vi "RFmxSpecAn Config per Harm & Freq Range (Harms).vi"(0 "SA Handle In":refnum<k21> caption="Instrument Handle In", 1 "# of Harms":u8, 7 "Center Freq (Hz) In":dbl, 11 "error in (no error)":errorcluster, 12 "Read Config File":bool, 13 "Meas Harm #":u8) -> (4 "SA Handle Out":refnum<k21> caption="Instrument Handle Out", 8 "Center Freq (Hz) Out":dbl, 15 "error out":errorcluster)   [LabVIEW 2018]
uses:
  Config Settings.ctl
  <vilib>/Utility/file.llb/Read Delimited Spreadsheet (string).vi
  <resource>/objmgr/RFmxInstr.rc
  <resource>/objmgr/RFmxSpecAn.rc
panel:
  out "Config Settings List":T1[][](array[typedef])
  out "Config Settings":T1
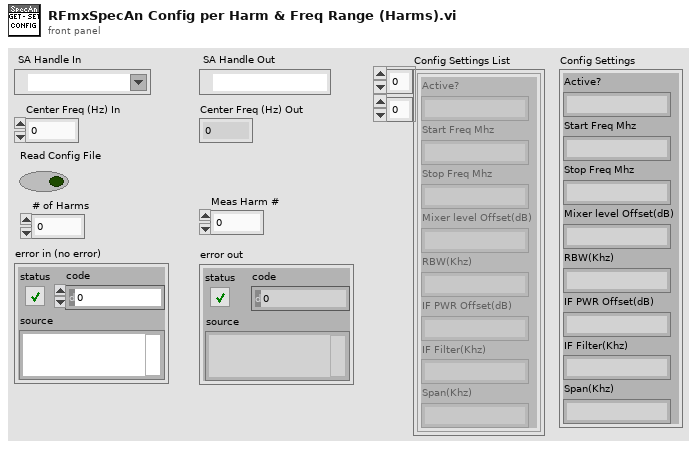
[diagram p1: front panel]
types:
  T1 = typedef "Config Settings.ctl" = cluster{"Active?":string, "Start Freq Mhz":string, "Stop Freq Mhz":string, "Mixer level Offset(dB)":string, "RBW(Khz)":string, "IF PWR Offset(dB)":string, "IF Filter(Khz)":string, "Span(Khz)":string}
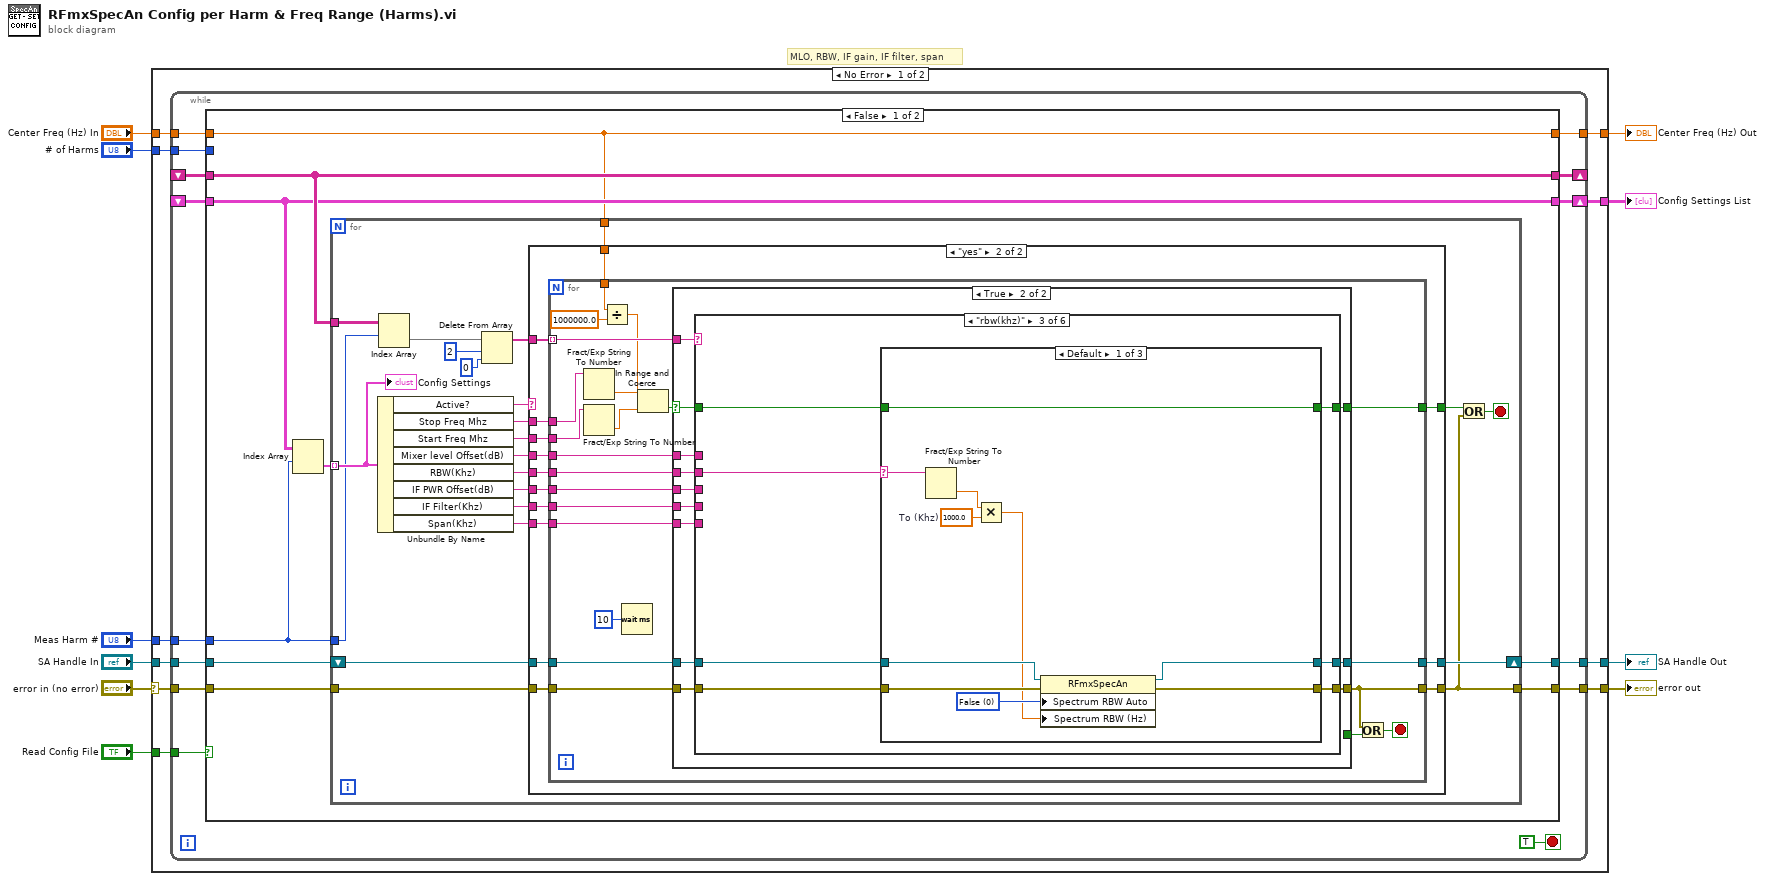
[diagram p0: block diagram]
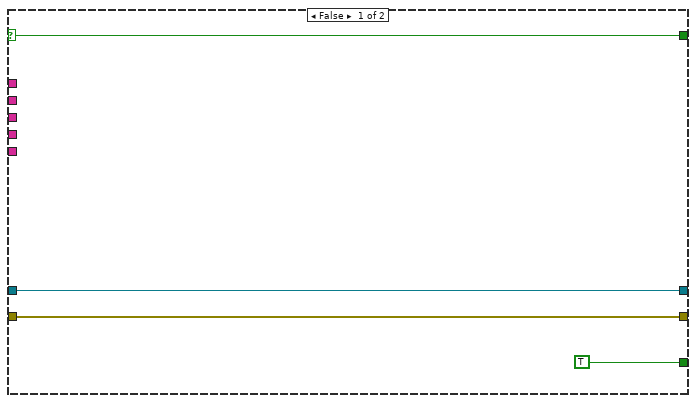
[diagram p3: hidden frame]
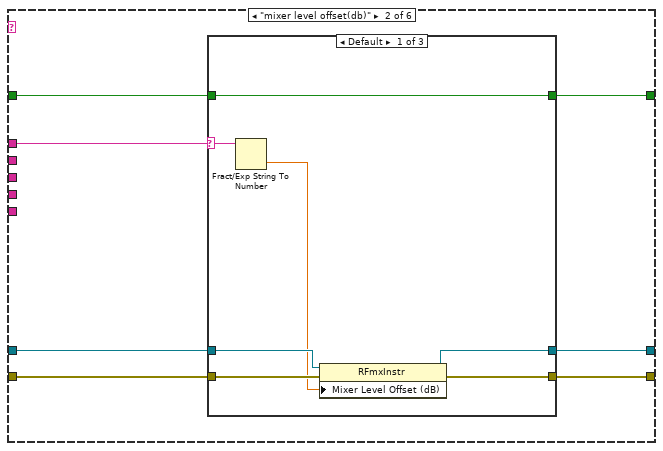
[diagram p5: hidden frame]
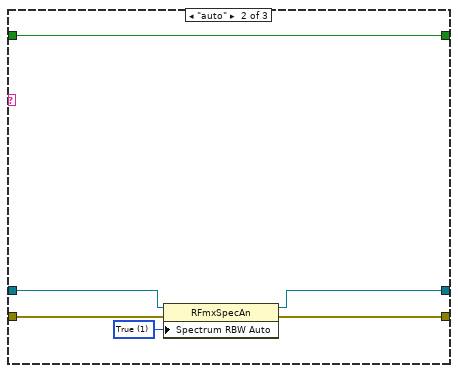
[diagram p8: hidden frame]
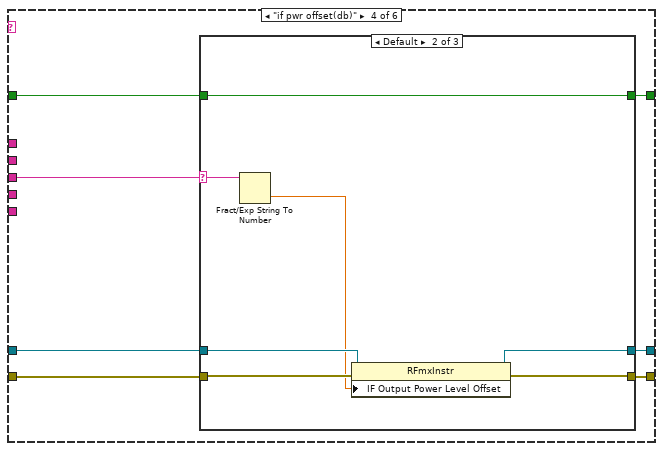
[diagram p10: hidden frame]
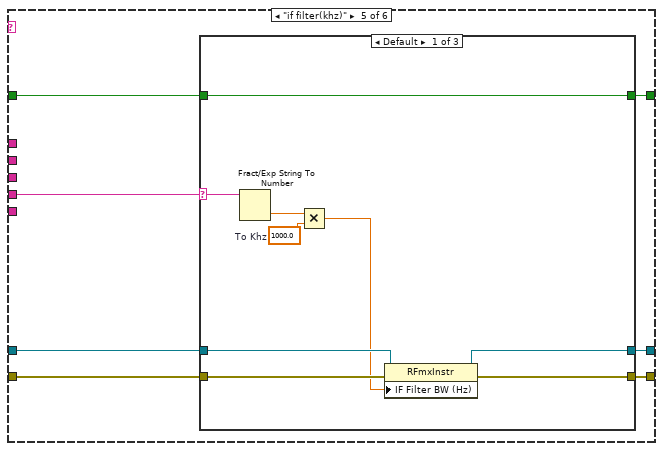
[diagram p13: hidden frame]
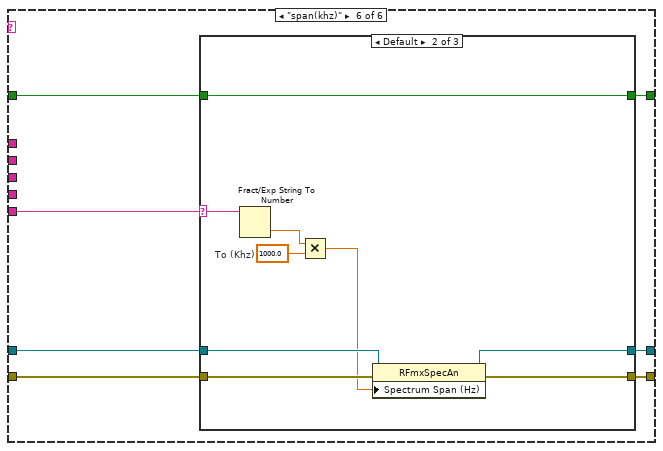
[diagram p16: hidden frame]
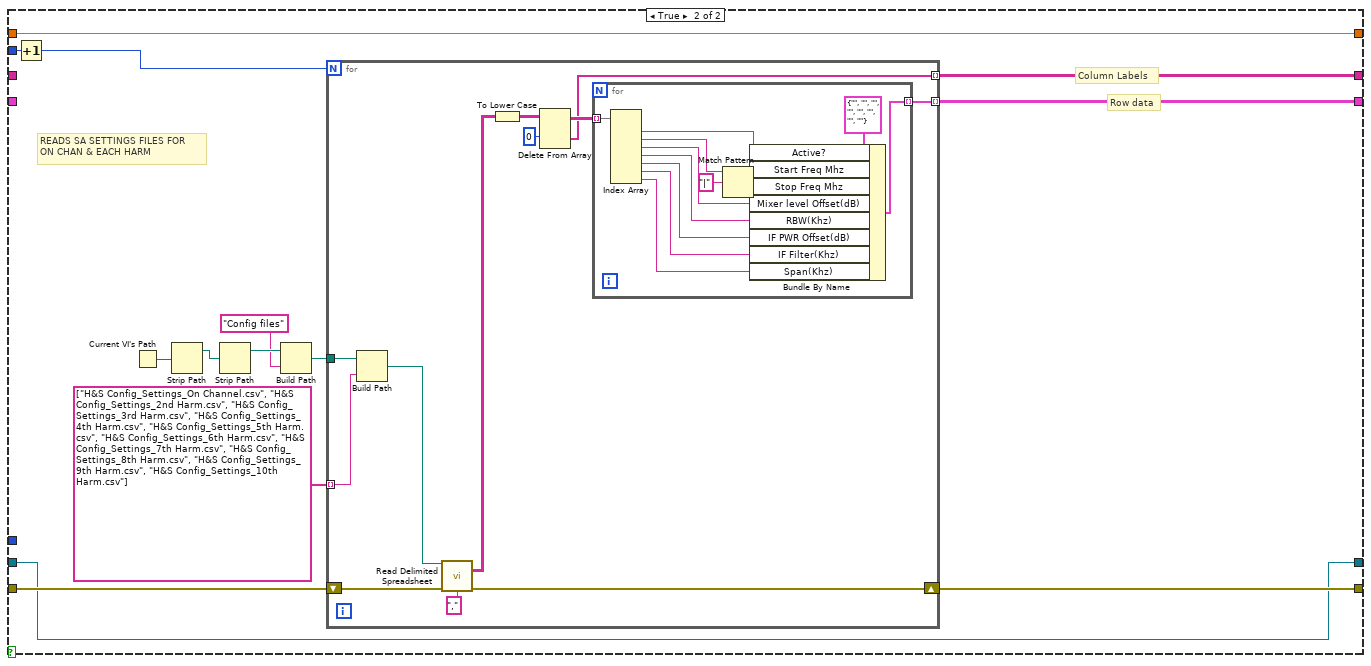
[diagram p19: hidden frame]
diagram:
  # "MLO, RBW, IF gain, IF filter, span"
  n1 = case shown="No Error" "error in (no error)" {
    selector: "error in (no error)" -> [w16 w274]
    tunnel: [w15 w274] -> w2
    tunnel: "SA Handle In" -> [w20 w273]
    tunnel: [w18 w273] -> w1
    tunnel: "Center Freq (Hz) In" -> [w19 w272]
    tunnel: [w17 w272] -> w8
    tunnel: [w14 _] -> w4
    tunnel: "Read Config File" -> [w13 _]
    tunnel: "Meas Harm #" -> [w12 _]
    tunnel: "# of Harms" -> [w11 _]
    frame No Error {
      n2 = while {
        tunnel: w20 -> [w24]
        tunnel: w19 -> [w28]
        tunnel: [w23] -> w18
        tunnel: [w27] -> w17
        tunnel: w16 -> [w33]
        tunnel: [w32] -> w15
        shift-right: [w31] -> w14
        shift-left: _ -> [w29]
        tunnel: w13 -> [w30]
        shift-right: [w26] -> _
        shift-left: _ -> [w25]
        tunnel: w12 -> [w22]
        tunnel: w11 -> [w21]
        stop <- TRUE stop-if-true
        n3 = case shown="False" w30 {
          tunnel: w33 -> [w43 w246]
          tunnel: [w36 w245] -> w32
          tunnel: [w41 w244] -> w31
          tunnel: w29 -> [w41 _]
          tunnel: w28 -> [w40 w243]
          tunnel: [w40 w243] -> w27
          tunnel: [w42 w242] -> w26
          tunnel: w25 -> [w42 _]
          tunnel: w24 -> [w39 w241]
          tunnel: [w35 w241] -> w23
          tunnel: w22 -> [w37 _]
          tunnel: w21 -> [_ w236]
          frame False {
            n4 = Index Array(array=w41, index (row)=w37) -> (element=w38:T1[])  [unwired: 1 in]
            n5 = for {
              tunnel: w42 -> [w64]
              tunnel: w40 -> [w63]
              tunnel: w38 -> [w52] mode=indexing
              tunnel: w37 -> [w50]
              shift-right: [w61] -> w35
              shift-left: w39 -> [w62]
              tunnel: w43 -> [w65]
              tunnel: [w45] -> w36
              stop <- w46 stop-if-true
              n6 = Unbundle By Name(w52) -> ("Active?"=w54:string, "Stop Freq Mhz"=w58:string, "Start Freq Mhz"=w57:string, "Mixer level Offset(dB)"=w56:string, "RBW(Khz)"=w55:string, "IF PWR Offset(dB)"=w49:string, "IF Filter(Khz)"=w48:string, "Span(Khz)"=w47:string)
              n7 = Index Array(array=w64, index (row)=w50) -> (element=w51:string[])  [unwired: 1 in]
              n8 = Delete From Array(array=w51, length=2, index=0) -> (array with subset deleted=w60:string[])  [unwired: 1 out]
              n9 = case shown="\"yes\"" w54 {
                tunnel: w65 -> [w67 w81]
                tunnel: [w67 w75] -> w45
                tunnel: w60 -> [_ w80]
                tunnel: w58 -> [_ w79]
                tunnel: w57 -> [_ w78]
                tunnel: w56 -> [_ w77]
                tunnel: w55 -> [_ w76]
                tunnel: w63 -> [_ w74]
                tunnel: [_ w73] -> w44
                tunnel: w62 -> [w66 w72]
                tunnel: [w66 w71] -> w61
                tunnel: w49 -> [_ w70]
                tunnel: w48 -> [_ w69]
                tunnel: w47 -> [_ w68]
                frame "no", Default {
                }
                frame "yes" {
                  n10 = for {
                    tunnel: w81 -> [w103]
                    tunnel: w80 -> [w102] mode=indexing
                    tunnel: w79 -> [w97]
                    tunnel: w78 -> [w96]
                    tunnel: w77 -> [w101]
                    tunnel: w76 -> [w100]
                    tunnel: [w86] -> w75
                    tunnel: w74 -> [w91]
                    tunnel: [w94] -> w73
                    tunnel: w72 -> [w93]
                    tunnel: [w92] -> w71
                    tunnel: w70 -> [w85]
                    tunnel: w69 -> [w84]
                    tunnel: w68 -> [w83]
                    stop <- w88 stop-if-true
                    n11 = Fract/Exp String To Number(string=w97) -> (number=w98:dbl)  [unwired: 3 in, 1 out]
                    n12 = Fract/Exp String To Number(string=w96) -> (number=w95:dbl)  [unwired: 3 in, 1 out]
                    n13 = Divide(x=w91, y=1000000.0) -> (x/y=w89:dbl)
                    n14 = Wait (ms)(milliseconds to wait=u32 10) -> ()  [unwired: 1 out]
                    n15 = In Range and Coerce(upper limit=w98, x=w89, lower limit=w95) -> (In Range?=w99:bool)  [unwired: 1 out]
                    n16 = case shown="True" w99 {
                      selector: w99 -> [w106 w114]
                      tunnel: w103 -> [w105 w119]
                      tunnel: w102 -> [_ w118]
                      tunnel: w101 -> [_ w117]
                      tunnel: w100 -> [_ w116]
                      tunnel: [w105 w115] -> w86
                      tunnel: [TRUE _] -> w87
                      tunnel: [w106 w113] -> w94
                      tunnel: w93 -> [w104 w112]
                      tunnel: [w104 w111] -> w92
                      tunnel: w85 -> [_ w110]
                      tunnel: w84 -> [_ w109]
                      tunnel: w83 -> [_ w108]
                      frame False {
                      }
                      frame True {
                        n17 = case shown="\"rbw(khz)\"" w118 {
                          tunnel: w119 -> [w121 w126 w147 w173 w193 w215]
                          tunnel: w117 -> [_ w127 _ _ _ _]
                          tunnel: w116 -> [_ _ w143 _ _ _]
                          tunnel: [w121 w125 w146 w172 w192 w214] -> w115
                          tunnel: w114 -> [w122 w129 w149 w175 w195 w217]
                          tunnel: [w122 w128 w148 w174 w194 w216] -> w113
                          tunnel: w112 -> [w120 w124 w145 w171 w191 w213]
                          tunnel: [w120 w123 w144 w170 w190 w212] -> w111
                          tunnel: w110 -> [_ _ _ w169 _ _]
                          tunnel: w109 -> [_ _ _ _ w189 _]
                          tunnel: w108 -> [_ _ _ _ _ w211]
                          frame "none", Default {
                          }
                          frame "mixer level offset(db)" {
                            n18 = case shown="Default" w127 {
                              selector: w127 -> [w131 _ _]
                              tunnel: w129 -> [w136 w139 w142]
                              tunnel: [w136 w139 w142] -> w128
                              tunnel: w126 -> [w135 w138 w141]
                              tunnel: [w133 w138 w141] -> w125
                              tunnel: w124 -> [w134 w137 w140]
                              tunnel: [w132 w137 w140] -> w123
                              frame Default {
                                n19 = Fract/Exp String To Number(string=w131) -> (number=w130:dbl)  [unwired: 3 in, 1 out]
                                n20 = property class="RFmxInstr"(reference=w134, error in=w135, "Mixer Level Offset (dB)"=w130) -> (reference out=w132:refnum<k21>, error out=w133:errorcluster)
                              }
                              frame "auto" {
                              }
                              frame "as found" {
                              }
                            }
                          }
                          frame "rbw(khz)" {
                            n21 = case shown="Default" w143 {
                              selector: w143 -> [w158 _ _]
                              tunnel: w149 -> [w159 w165 w168]
                              tunnel: [w159 w165 w168] -> w148
                              tunnel: w147 -> [w157 w164 w166]
                              tunnel: [w156 w163 w166] -> w146
                              tunnel: w145 -> [w154 w161 w167]
                              tunnel: [w155 w162 w167] -> w144
                              frame Default {
                                w150 = 1000.0  # To (Khz)
                                w153 = 0 items=["False", "True"] ("Spectrum RBW Auto")
                                n22 = Fract/Exp String To Number(string=w158) -> (number=w152:dbl)  [unwired: 3 in, 1 out]
                                n23 = Multiply(x=w152, y=w150) -> (x*y=w151:dbl)
                                n24 = property class="RFmxSpecAn"(reference=w154, error in=w157, "Spectrum RBW Auto"=w153, "Spectrum RBW (Hz)"=w151) -> (reference out=w155:refnum<k21>, error out=w156:errorcluster)
                              }
                              frame "auto" {
                                w160 = 1 items=["False", "True"] ("Spectrum RBW Auto")
                                n25 = property class="RFmxSpecAn"(reference=w161, error in=w164, "Spectrum RBW Auto"=w160) -> (reference out=w162:refnum<k21>, error out=w163:errorcluster)
                              }
                              frame "as found" {
                              }
                            }
                          }
                          frame "if pwr offset(db)" {
                            n26 = case shown="Default" w169 {
                              selector: w169 -> [_ w184 _]
                              tunnel: w175 -> [w178 w185 w188]
                              tunnel: [w178 w185 w188] -> w174
                              tunnel: w173 -> [w176 w183 w186]
                              tunnel: [w176 w181 w186] -> w172
                              tunnel: w171 -> [w177 w182 w187]
                              tunnel: [w177 w180 w187] -> w170
                              frame "auto" {
                              }
                              frame Default {
                                n27 = Fract/Exp String To Number(string=w184) -> (number=w179:dbl)  [unwired: 3 in, 1 out]
                                n28 = property class="RFmxInstr"(reference=w182, error in=w183, "IF Output Power Level Offset"=w179) -> (reference out=w180:refnum<k21>, error out=w181:errorcluster)
                              }
                              frame "as found" {
                              }
                            }
                          }
                          frame "if filter(khz)" {
                            n29 = case shown="Default" w189 {
                              selector: w189 -> [w203 _ _]
                              tunnel: w195 -> [w204 w207 w210]
                              tunnel: [w204 w207 w210] -> w194
                              tunnel: w193 -> [w202 w205 w208]
                              tunnel: [w201 w205 w208] -> w192
                              tunnel: w191 -> [w200 w206 w209]
                              tunnel: [w199 w206 w209] -> w190
                              frame Default {
                                w196 = 1000.0  # To Khz
                                n30 = Fract/Exp String To Number(string=w203) -> (number=w197:dbl)  [unwired: 3 in, 1 out]
                                n31 = Multiply(x=w197, y=w196) -> (x*y=w198:dbl)
                                n32 = property class="RFmxInstr"(reference=w200, error in=w202, "IF Filter BW (Hz)"=w198) -> (reference out=w199:refnum<k21>, error out=w201:errorcluster)
                              }
                              frame "auto" {
                              }
                              frame "as found" {
                              }
                            }
                          }
                          frame "span(khz)" {
                            n33 = case shown="Default" w211 {
                              selector: w211 -> [_ w228 _]
                              tunnel: w217 -> [w220 w229 w232]
                              tunnel: [w220 w229 w232] -> w216
                              tunnel: w215 -> [w218 w226 w230]
                              tunnel: [w218 w225 w230] -> w214
                              tunnel: w213 -> [w219 w227 w231]
                              tunnel: [w219 w224 w231] -> w212
                              frame "auto" {
                              }
                              frame Default {
                                w221 = 1000.0  # To (Khz)
                                n34 = Fract/Exp String To Number(string=w228) -> (number=w222:dbl)  [unwired: 3 in, 1 out]
                                n35 = Multiply(x=w222, y=w221) -> (x*y=w223:dbl)
                                n36 = property class="RFmxSpecAn"(reference=w227, error in=w226, "Spectrum Span (Hz)"=w223) -> (reference out=w224:refnum<k21>, error out=w225:errorcluster)
                              }
                              frame "as found" {
                              }
                            }
                          }
                        }
                      }
                    }
                    n37 = Or(x=w86, y=w87) -> (x .or. y?=w88:bool)
                  }
                }
              }
              n38 = Or(x=w44, y=w45) -> (x .or. y?=w46:bool)
              "Config Settings" <- w52
            }
          }
          frame True {
            # "READS SA SETTINGS FILES FOR \nON CHAN & EACH HARM"
            # "Row data"
            # "Column Labels"
            n39 = Increment(x=w236) -> (x+1=w235:u8)
            n40 = Current VI's Path() -> (path=w234:path)
            n41 = Strip Path(path=w234) -> (stripped path=w233:path)  [unwired: 1 out]
            n42 = Strip Path(path=w233) -> (stripped path=w239:path)  [unwired: 1 out]
            n43 = Build Path(base path=w239, name or relative path="Config files") -> (appended path=w238:path)
            n44 = for {
              N: w235 -> [_]
              tunnel: [w255] -> w244 mode=indexing
              tunnel: [w251] -> w242 mode=indexing
              shift-right: [w257] -> w245
              shift-left: w246 -> [w258]
              tunnel: string[] ["H&S Config_Settings_On Channel.csv", "H&S Config_Settings_2nd Harm.csv", "H&S Config_Settings_3rd Harm.csv", "H&S Config_Settings_4th Harm.csv", "H&S Config_Settings_5th Harm.csv", "H&S Config_Settings_6th Harm.csv", "H&S Config_Settings_7th Harm.csv", "H&S Config_Settings_8th Harm.csv", "H&S Config_Settings_9th Harm.csv", "H&S Config_Settings_10th Harm.csv"] -> [w248] mode=indexing
              tunnel: w238 -> [w249]
              n45 = Build Path(base path=w249, name or relative path=w248) -> (appended path=w247:path)
              n46 = call-poly <vilib>:"Read Delimited Spreadsheet.vi"("file path (dialog if empty)"=w247, "error in (no error)"=w258, "delimiter (\\t)"="," ("delimiter (\\t)")) -> ("all rows"=w254:string[][], "error out"=w257:errorcluster)  [unwired: 7 in, 4 out]
              n47 = To Lower Case(string=w254) -> (all lower case string=w250:string[][])
              n48 = Delete From Array(array=w250, index (row)=0) -> (deleted portion=w251:string[], array with subset deleted=w252:string[][])  [unwired: 2 in]
              n49 = for {
                tunnel: w252 -> [w271] mode=indexing
                tunnel: [w266] -> w255 mode=indexing
                n50 = Index Array(array=w271) -> (element #1=w265:string, element #2=w264:string, element #3=w263:string, element #4=w262:string, element #5=w261:string, element #6=w260:string, element #7=w259:string)  [unwired: 7 in]
                n51 = Match Pattern(string=w264, regular expression="|") -> (before substring=w268:string, after substring=w267:string)  [unwired: 1 in, 2 out]
                n52 = Bundle By Name(cluster=T1 {"Active?"="", "Start Freq Mhz"="", "Stop Freq Mhz"="", "Mixer level Offset(dB)"="", "RBW(Khz)"="", "IF PWR Offset(dB)"="", "IF Filter(Khz)"="", "Span(Khz)"=""} ("Config Settings"), "Active?"=w265, "Start Freq Mhz"=w268, "Stop Freq Mhz"=w267, "Mixer level Offset(dB)"=w263, "RBW(Khz)"=w262, "IF PWR Offset(dB)"=w261, "IF Filter(Khz)"=w260, "Span(Khz)"=w259) -> (w266:T1)
              }
            }
          }
        }
      }
    }
    frame Error {
    }
  }
  "error out" <- w2
  "Center Freq (Hz) Out" <- w8
  "SA Handle Out" <- w1
  "Config Settings List" <- w4
